vi "Append To Dataset 1D Integer.vi"(8 "error in (no error)":errorcluster, 10 "data":i32[](array[numeric]), 11 "Dataset id in":i32) -> (0 "Error out":errorcluster, 3 "Dataset id out":i32)   [LabVIEW 2014]
uses:
  HDF5Tools.lvlib
  Release/HDF5Tools.dll
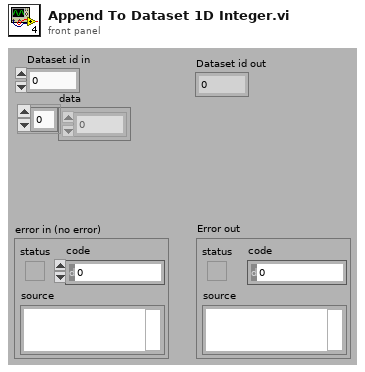
[diagram p1: front panel]
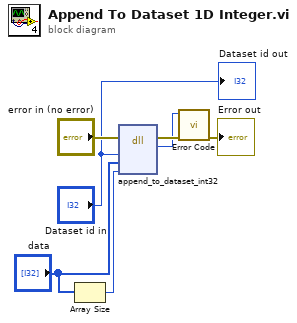
[diagram p0: block diagram]
diagram:
  n1 = Array Size(array="data") -> (size(s)=w2:i32)
  n2 = dll-call lib="C:/HDF5Tools/Release/HDF5Tools.dll" fn="append_to_dataset_int32"(error in="error in (no error)", "dataset_id"="Dataset id in", "data"="data", "count"=w2) -> (error out=w5:errorcluster, "error"=w3:i32)  [unwired: 5 in, 1 out]
  n3 = call "Error Code.vi"("Error in"=w5, "Error code"=w3) -> ("Error out"=→"Error out":errorcluster)  [unwired: 9 in]
  "Dataset id out" <- "Dataset id in"
